vi "Test Server API.vi"() -> ()   [LabVIEW 2019]
doc: "Server API Tester."
uses:
  TypeDef/ISO.ctl
  TypeDef/Noise.ctl
  TypeDef/Link.ctl
  TypeDef/Sett data.ctl
  Server.lvlib
  Setting Panel/Setting Panel.lvlib
panel:
  out "Distance 2":dbl
  out "Signal gain 2":dbl
  out "Noise attenuator 2":dbl
  out "Link 2":T1
  out "Type noise 2":T2
  out "M 2":cluster{"Метка":i64, "Считыветель":i64}
  out "BM 3":cluster{"R":dbl, "C":dbl, "L":dbl}
  out "BI 3":cluster{"R":dbl, "C":dbl, "L":dbl}
  out "ISO/IEC w 2":T3
  out "Bit rate 3":dbl
  out "Gain 2":dbl
  out "Filter 3":i32
  out "Distance":dbl
  out "Signal gain":dbl
  out "Noise attenuator":dbl
  out "Link":T1
  out "Type noise":T2
  out "M":cluster{"Метка":i64, "Считыветель":i64}
  out "BM 2":cluster{"R":dbl, "C":dbl, "L":dbl}
  out "BI 2":cluster{"R":dbl, "C":dbl, "L":dbl}
  out "ISO/IEC w":T3
  out "Bit rate 2":dbl
  out "Gain":dbl
  out "Filter 2":i32
  in  "Bit rate":dbl=32.0 min=4.0 max=128.0 step=4.0
  in  "Filter":i32=3 min=1 max=15 step=1
  in  "Type noise w":T2
  in  "M w":cluster{"Метка":i64, "Считыветель":i64}={"Метка"=10, "Считыветель"=100} {"Считыветель" min=10 max=10 step=100; "Метка" min=10 max=10 step=100}
  in  "BM":cluster{"R":dbl, "C":dbl, "L":dbl}={"R"=1.0, "C"=0.01, "L"=1e-05} {"L" min=1e-05 max=1.5e-05 step=1e-06 format="%#_6p"; "C" min=0.01 max=0.15 step=0.001 format="%#_6p"; "R" min=1.0 max=150.0 step=1.0 format="%#_6p"}
  in  "BI":cluster{"R":dbl, "C":dbl, "L":dbl}={"R"=1.0, "C"=0.01, "L"=1e-05} {"L" min=1e-05 max=1.5e-05 step=1e-06 format="%#_6p"; "C" min=0.01 max=0.15 step=0.001 format="%#_6p"; "R" min=1.0 max=150.0 step=1.0 format="%#_6p"}
  in  "Иммитатор расстояния":dbl(slide)=3.0 min=3.0 max=1500.0 step=1.0 scale=3.0..1500.0
  in  "Усилитель сигнала":dbl(knob)=1.0 min=1.0 max=100.0 step=1.0 scale=1.0..30.0
  in  "Выбор стандарта":T3
  in  "Аттенюатор шума":dbl(knob)=1.0 min=1.0 max=10.0 step=0.1 scale=1.0..30.0
  in  "Apply Settings":bool
  in  "wait for reply":bool=TRUE
  in  "Show Block Diagram":bool
  in  "X":dbl=1.0
  out "Reply Payload":dbl
  in  "Stop Module":bool
  in  "Start Module":bool
  out "Do Something Count":i32
  in  "Test Do Something Else and Wait for Reply":bool
  in  "Hide Module Panel":bool
  in  "Show Module Panel":bool
  in  "Test Do Something Else":bool
  in  "Start":bool
  out "Status":string
  out "Module Running?":bool
  # "Данные отправляемые в модуль"
  # "Данные из модуля\n Settings"
  # "При нажатии кнопки Apply на лицевой\nпанели модуля Server"
  # "This VI tests the API for the Module."
  # "БУПУЭМСС"
  # "БУПУЭМСМ"
  # "Коэффициент модуляции, %"
  # "Скорость"
  # "Порядок фильтра"
  # "Для отправления данных в модули\nработчих каналов"
  # "мм"
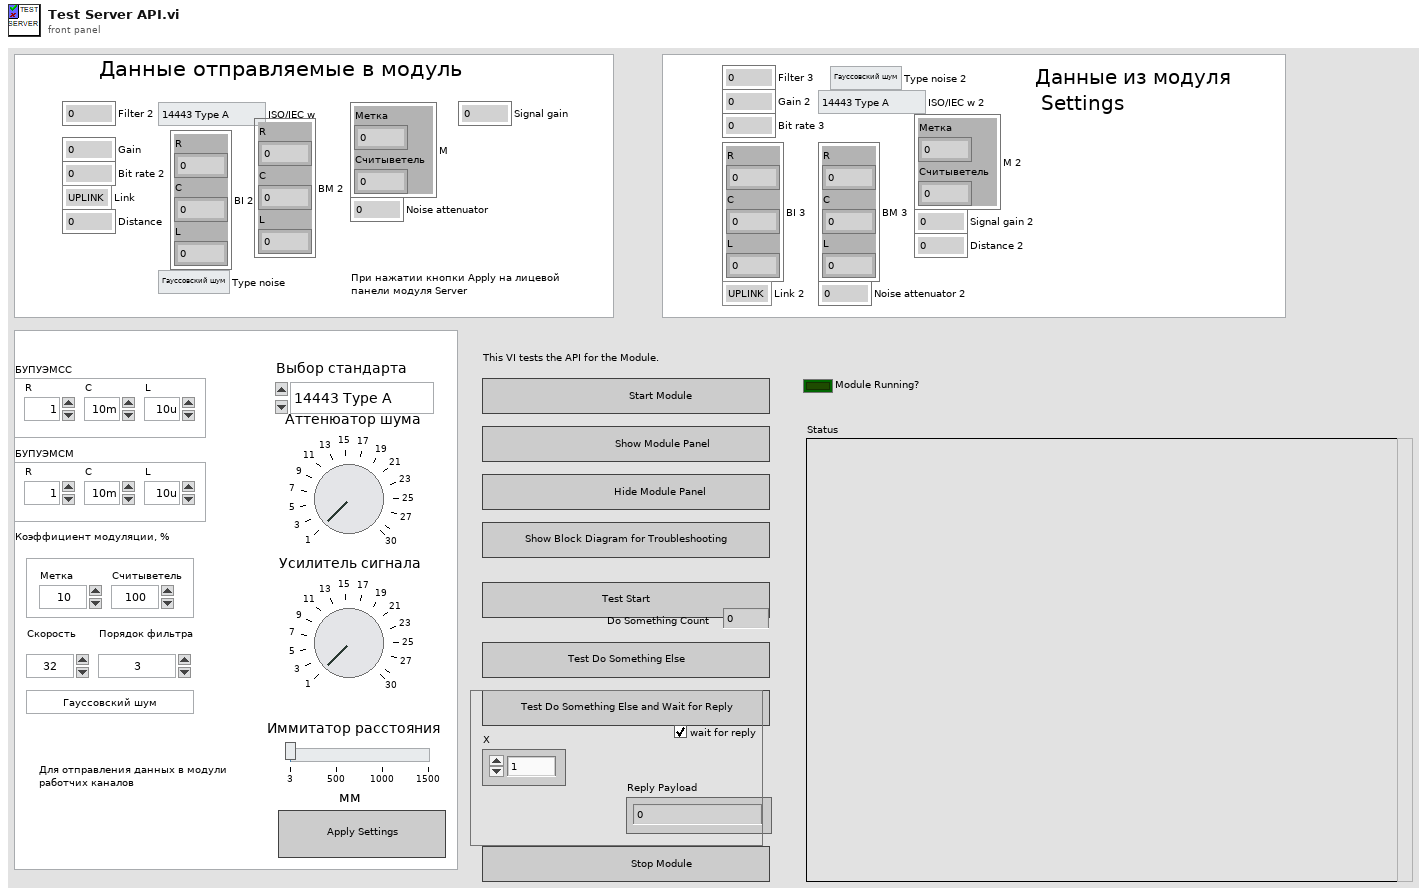
[diagram p1: front panel]
types:
  T1 = typedef "Link.ctl" = enum16{"UPLINK", "DOWNLINK"}
  T2 = typedef "Noise.ctl" = enum16{"Гауссовский шум", "Белый шум"}
  T3 = typedef "ISO.ctl" = enum16{"14443 Type A", "14443 Type B", "Felica", "15693"}
  T4 = typedef "Server.lvlib/Broadcast Events--cluster.ctl" = cluster{"Module Did Init":refnum<user-event>, "Status Updated":refnum<user-event>, "Error Reported":refnum<user-event>, "Did Something":refnum<user-event>, "Module Did Stop":refnum<user-event>, "Update Module Execution Status":refnum<user-event>, "Apply settings":refnum<user-event>}
  T5 = typedef "Setting Panel.lvlib/Broadcast Events--cluster.ctl" = cluster{"Module Did Init":refnum<user-event>, "Status Updated":refnum<user-event>, "Error Reported":refnum<user-event>, "Did Something":refnum<user-event>, "Module Did Stop":refnum<user-event>, "Update Module Execution Status":refnum<user-event>, "Get data":refnum<user-event>}
  T6 = typedef "Sett data.ctl" = cluster{"Filter":i32, "Gain":dbl, "Bit rate":dbl, "ISO/IEC w ":T3, "BI":cluster{"R":dbl, "C":dbl, "L":dbl}, "BM":cluster{"R":dbl, "C":dbl, "L":dbl}, "M":cluster{"Метка":i64, "Считыветель":i64}, "Type noise":T2, "Link":T1, "Noise attenuator":dbl, "Signal gain":dbl, "Distance":dbl}
  T7 = typedef "Server.lvlib/Do Something Else and Wait (Reply Payload)--cluster.ctl" = cluster{"Value":dbl, "error":errorcluster}
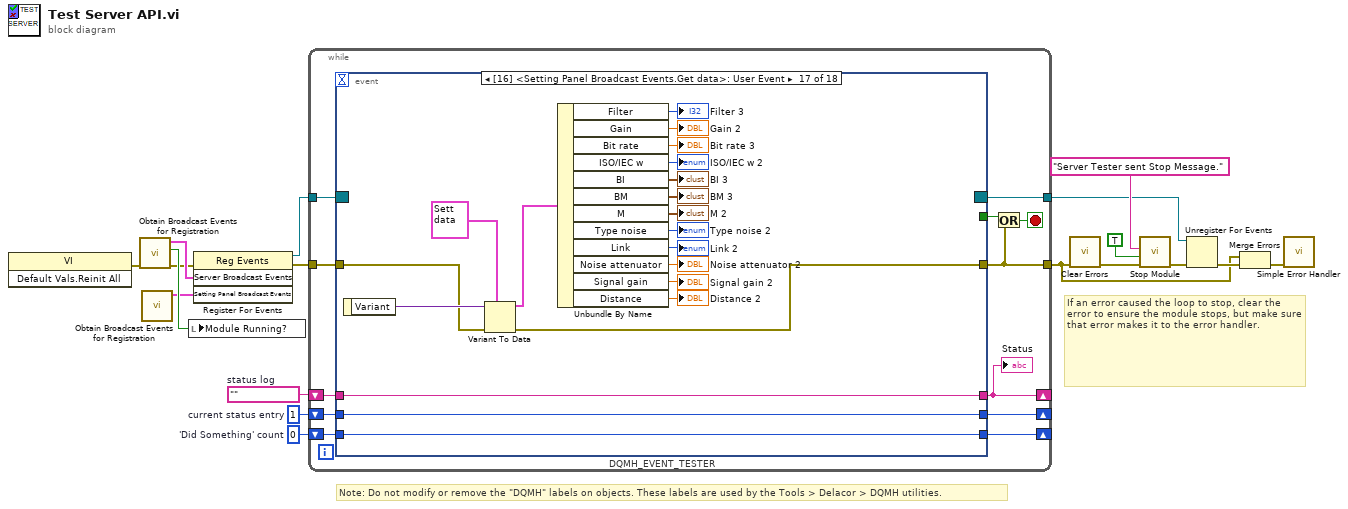
[diagram p0: block diagram]
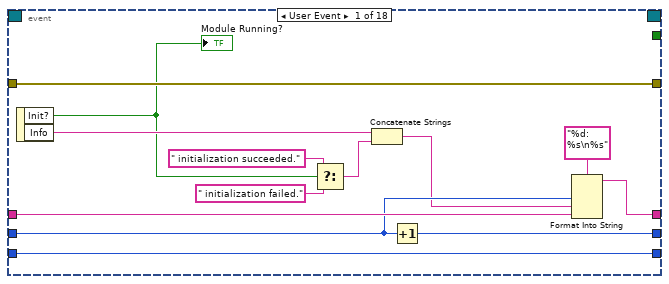
[diagram p2: hidden frame]
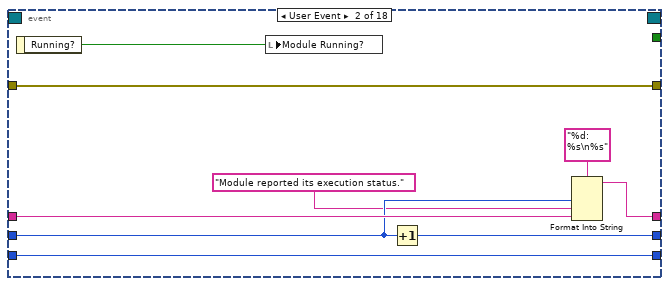
[diagram p3: hidden frame]
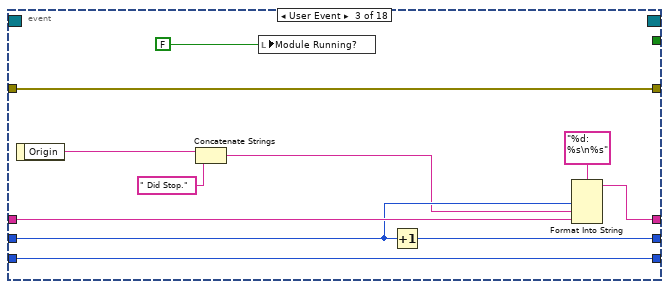
[diagram p4: hidden frame]
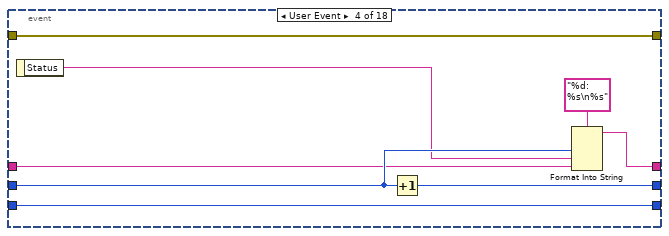
[diagram p5: hidden frame]
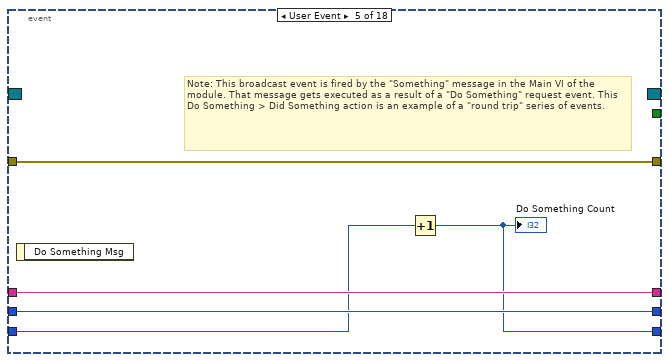
[diagram p6: hidden frame]
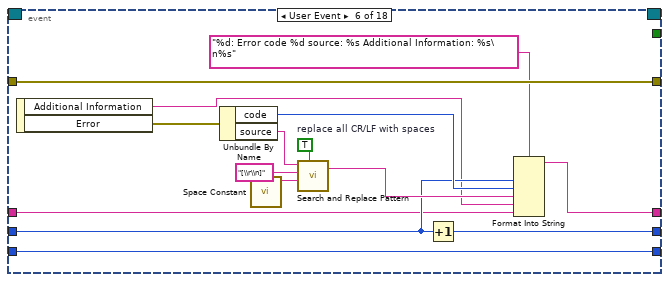
[diagram p7: hidden frame]
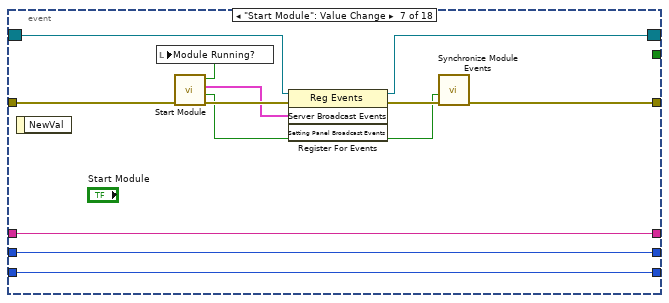
[diagram p8: hidden frame]
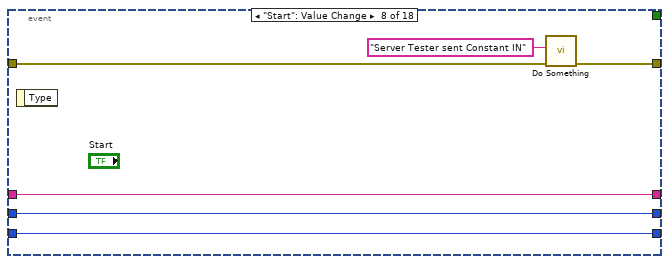
[diagram p9: hidden frame]
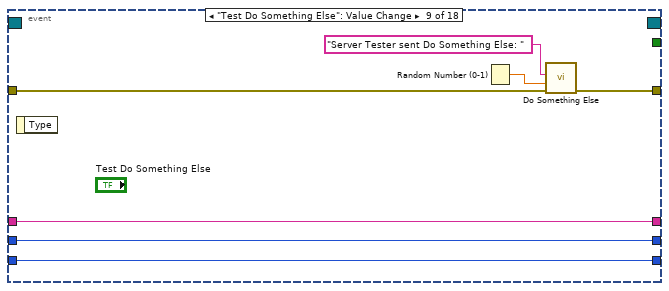
[diagram p10: hidden frame]
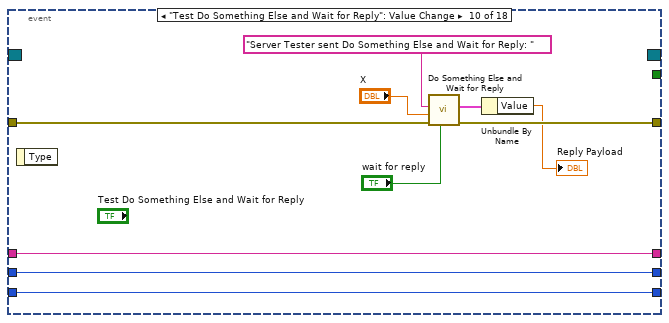
[diagram p11: hidden frame]
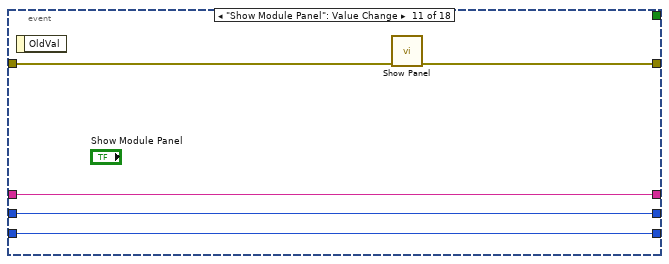
[diagram p12: hidden frame]
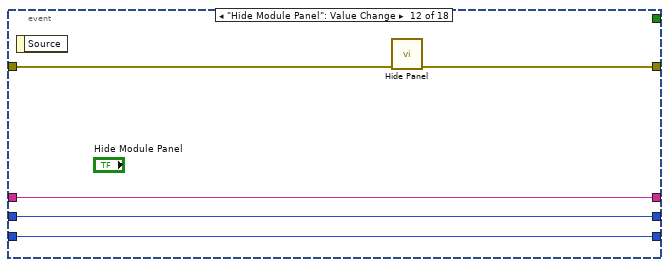
[diagram p13: hidden frame]
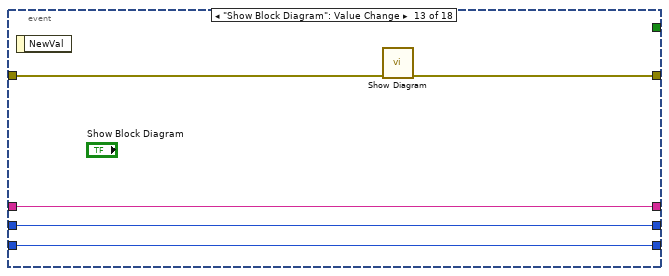
[diagram p14: hidden frame]
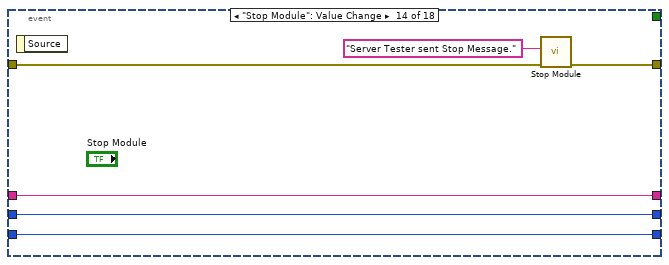
[diagram p15: hidden frame]
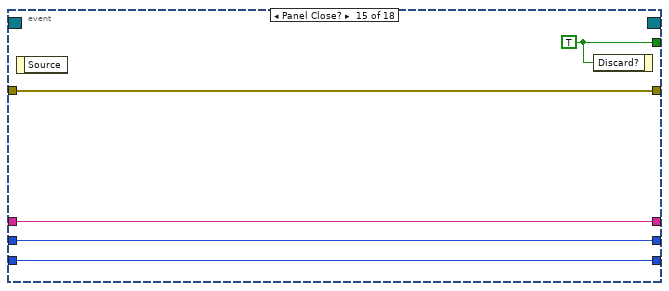
[diagram p16: hidden frame]
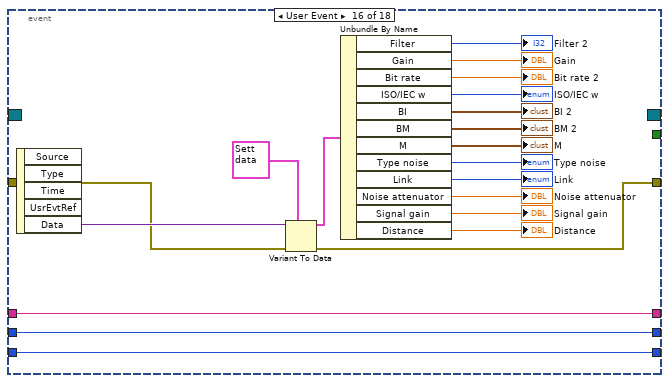
[diagram p17: hidden frame]
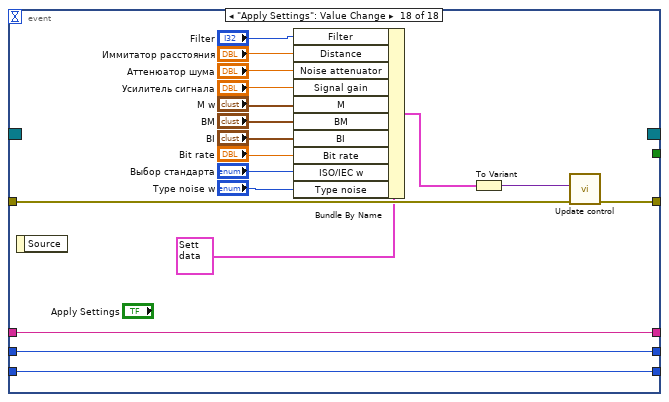
[diagram p18: hidden frame]
diagram:
  w13 = 0  # 'Did Something' count
  w14 = 1  # current status entry
  w15 = ""  # status log
  # "If an error caused the loop to stop, clear the error to ensure the module stops, but make sure that error makes it to the error handler."
  # "Note: Do not modify or remove the \"DQMH\" labels on objects. These labels are used by the Tools > Delacor > DQMH utilities."
  n1 = invoke class="VI" method="Default Vals.Reinit All"() -> (error out=w3:errorcluster)  [unwired: 3 in, 2 out]
  n2 = call "Obtain Broadcast Events for Registration.vi"("error in (no error)"=w3) -> ("error out"=w2:errorcluster, "Already running?"=w4:bool, "Server Broadcast Events"=w11:T4)  [unwired: 8 in]
  n3 = call "Obtain Broadcast Events for Registration.vi"() -> ("Setting Panel Broadcast Events"=w1:T5)  [unwired: 9 in, 2 out]
  n4 = local write "Module Running?"(w4) -> ()
  n5 = register-events(error in=w2, w11, w1) -> (reference out=w10:refnum<event-registration>, error out=w12:errorcluster)  [unwired: 1 in]
  n6 = while {
    tunnel: w10 -> [w30]
    tunnel: [w19] -> w5
    shift-right: [w25] -> _
    shift-left: w15 -> [w27]
    shift-right: [w26] -> _
    shift-left: w14 -> [w28]
    shift-right: [w23] -> _
    shift-left: w13 -> [w24]
    tunnel: w12 -> [w21]
    tunnel: [w20] -> w9
    stop <- w22 stop-if-true
    n7 = event "DQMH_EVENT_TESTER" shown="[16] <Setting Panel Broadcast Events.Get data>: User Event" {
      selector: w30 -> [_ _ _ _ _ _ w96 _ _ _ _ _ _ _ _ _ _ _]
      dyn-events: [_ _ _ _ _ _ w95 _ _ _ _ _ _ _ _ _ _ _] -> w20
      timeout: _ -> [_ _ _ _ _ _ _ _ _ _ _ _ _ _ _ _ _ _]
      tunnel: [_ _ _ _ _ _ _ _ _ _ _ _ _ _ w152 _ _ _] -> w29
      tunnel: [w43 w45 w53 w64 w72 w90 w94 w109 w116 w126 w131 w136 w137 w144 w148 w167 w187 w206] -> w19
      tunnel: w28 -> [w40 w50 w61 w68 w75 w80 w100 w106 w112 w123 w129 w134 w139 w146 w150 w171 w191 w208]
      tunnel: w27 -> [w41 w51 w62 w67 w76 w78 w101 w107 w113 w124 w130 w135 w140 w147 w151 w172 w192 w209]
      tunnel: [w38 w48 w59 w69 w76 w81 w101 w107 w113 w124 w130 w135 w140 w147 w151 w172 w192 w209] -> w25
      tunnel: [w39 w49 w60 w71 w75 w79 w100 w106 w112 w123 w129 w134 w139 w146 w150 w171 w191 w208] -> w26
      tunnel: w24 -> [w35 w46 w55 w65 w74 w91 w99 w105 w111 w122 w128 w133 w138 w145 w149 w170 w190 w207]
      tunnel: [w35 w46 w55 w65 w73 w91 w99 w105 w111 w122 w128 w133 w138 w145 w149 w170 w190 w207] -> w23
      tunnel: w21 -> [w43 w45 w53 w64 w72 w90 w93 w104 w110 w119 w127 w132 w141 w142 w148 w168 w188 w210]
      event User Event {
        n8 = event-data() -> ("Init?"=w34:bool, "Info"=w37:string)  [unwired: 1 in]
        "Module Running?" <- w34
        n9 = Select(t=" initialization succeeded.", s=w34, f=" initialization failed.") -> (s? t:f=w31:string)
        n10 = Concatenate Strings(w37, w31) -> (w36:string)
        n11 = Increment(x=w40) -> (x+1=w39:i32)
        n12 = Format Into String(format string="%d: %s\n%s", w40, w36, w41) -> (resulting string=w38:string)  [unwired: 2 in, 1 out]
      }
      event User Event {
        n13 = event-data() -> ("Running?"=w44:bool)  [unwired: 1 in]
        n14 = local write "Module Running?"(w44) -> ()
        n15 = Increment(x=w50) -> (x+1=w49:i32)
        n16 = Format Into String(format string="%d: %s\n%s", w50, "Module reported its execution status.", w51) -> (resulting string=w48:string)  [unwired: 2 in, 1 out]
      }
      event User Event {
        n17 = event-data() -> ("Origin"=w58:string)  [unwired: 1 in]
        n18 = Concatenate Strings(w58, " Did Stop.") -> (w57:string)
        n19 = local write "Module Running?"(FALSE ("Module Did Init?")) -> ()
        n20 = Increment(x=w61) -> (x+1=w60:i32)
        n21 = Format Into String(format string="%d: %s\n%s", w61, w57, w62) -> (resulting string=w59:string)  [unwired: 2 in, 1 out]
      }
      event User Event {
        n22 = event-data() -> ("Status"=w66:string)  [unwired: 1 in]
        n23 = Increment(x=w68) -> (x+1=w71:i32)
        n24 = Format Into String(format string="%d: %s\n%s", w68, w66, w67) -> (resulting string=w69:string)  [unwired: 2 in, 1 out]
      }
      event User Event {
        # "Note: This broadcast event is fired by the \"Something\" message in the Main VI of the module. That message gets executed as a result of a \"Do Something\" request event. This Do Something > Did Something action is an example of a \"round trip\" series of events."
        n25 = event-data() -> ()  [unwired: 1 in, 1 out]
        n26 = Increment(x=w74) -> (x+1=w73:i32)
        "Do Something Count" <- w73
      }
      event User Event {
        w86 = TRUE  # replace all CR/LF with spaces
        n27 = event-data() -> ("Additional Information"=w77:string, "Error"=w82:errorcluster)  [unwired: 1 in]
        n28 = Unbundle By Name(w82) -> ("code"=w83:i32, "source"=w84:string)
        n29 = call <vilib>:"Space Constant.vi"() -> ("String"=w87:string)
        n30 = call <vilib>:"Search and Replace Pattern.vi"("string"=w84, "regular expression (\"\")"="[\\r\\n]" ("regular expression (\"\")"), "replace string (\"\")"=w87, "replace all? (F)"=w86) -> ("result string"=w85:string)  [unwired: 1 in, 1 out]
        n31 = Increment(x=w80) -> (x+1=w79:i32)
        n32 = Format Into String(format string="%d: Error code %d source: %s Additional Information: %s\n%s", w80, w83, w85, w77, w78) -> (resulting string=w81:string)  [unwired: 2 in, 1 out]
      }
      event "Start Module": Value Change {
        n33 = event-data() -> ()  [unwired: 1 in, 1 out]
        n34 = call "Start Module.vi"("error in (no error)"=w93) -> ("error out"=w102:errorcluster, "Wait for Event Sync?"=w98:bool, "Server Broadcast Events"=w97:T4, "Module Was Already Running?"=w92:bool)  [unwired: 7 in]
        n35 = local write "Module Running?"(w92) -> ()
        n36 = register-events(reference=w96, error in=w102, w97) -> (reference out=w95:refnum<event-registration>, error out=w103:errorcluster)  [unwired: 1 in]
        n37 = call "Synchronize Module Events.vi"("error in (no error)"=w103, "Wait for Event Sync?"=w98) -> ("error out"=w94:errorcluster)  [unwired: 9 in]
      }
      event "Start": Value Change {
        n38 = event-data() -> ()  [unwired: 1 in, 1 out]
        n39 = call "Do Something.vi"("error in (no error)"=w104, "Do Something Message"="Server Tester sent Constant IN") -> ("error out"=w109:errorcluster)  [unwired: 9 in]
      }
      event "Test Do Something Else": Value Change {
        n40 = event-data() -> ()  [unwired: 1 in, 1 out]
        n41 = Random Number (0-1)() -> (number: 0 to 1=w114:dbl)
        n42 = call "Do Something Else.vi"("error in (no error)"=w110, "X"=w114, "Do Something Else Message"="Server Tester sent Do Something Else: " ("Do Something Message")) -> ("error out"=w116:errorcluster)  [unwired: 8 in]
      }
      event "Test Do Something Else and Wait for Reply": Value Change {
        n43 = event-data() -> ()  [unwired: 1 in, 1 out]
        n44 = call "Do Something Else and Wait for Reply.vi"("wait for reply (T)"="wait for reply", "error in (no error)"=w119, "X"="X", "Do Something Else Message"="Server Tester sent Do Something Else and Wait for Reply: " ("Do Something Message")) -> ("error out"=w126:errorcluster, "Reply Payload"=w121:T7)  [unwired: 5 in, 1 out]
        n45 = Unbundle By Name(w121) -> ("Value"=→"Reply Payload":dbl)
      }
      event "Show Module Panel": Value Change {
        n46 = event-data() -> ()  [unwired: 1 in, 1 out]
        n47 = call "Show Panel.vi"("error in (no error)"=w127) -> ("error out"=w131:errorcluster)  [unwired: 10 in]
      }
      event "Hide Module Panel": Value Change {
        n48 = event-data() -> ()  [unwired: 1 in, 1 out]
        n49 = call "Hide Panel.vi"("error in (no error)"=w132) -> ("error out"=w136:errorcluster)  [unwired: 10 in]
      }
      event "Show Block Diagram": Value Change {
        n50 = event-data() -> ()  [unwired: 1 in, 1 out]
        n51 = call "Show Diagram.vi"("error in (no error)"=w141) -> ("error out"=w137:errorcluster)  [unwired: 10 in]
      }
      event "Stop Module": Value Change {
        n52 = event-data() -> ()  [unwired: 1 in, 1 out]
        n53 = call "Stop Module.vi"("error in (no error)"=w142, "Origin"="Server Tester sent Stop Message.") -> ("error out"=w144:errorcluster)  [unwired: 9 in]
      }
      event Panel Close? {
        w152 = TRUE ("Discard?")
        n54 = event-data() -> ()  [unwired: 1 in, 1 out]
        n55 = event-data("Discard?"=w152) -> ()  [unwired: 1 in, 1 out]
      }
      event User Event {
        n56 = event-data() -> ("Data"=w169:variant)  [unwired: 1 in, 4 out]
        n57 = Variant To Data(error in=w168, type=T6 {"Filter"=0, "Gain"=0.0, "Bit rate"=0.0, "ISO/IEC w "=enum."14443 Type A", "BI"={"R"=0.0, "C"=0.0, "L"=0.0}, "BM"={"R"=0.0, "C"=0.0, "L"=0.0}, "M"={"Метка"=10, "Считыветель"=10}, "Type noise"=enum."Гауссовский шум", "Link"=enum."UPLINK", "Noise attenuator"=0.0, "Signal gain"=1.0, "Distance"=0.0} ("Sett data"), Variant=w169) -> (data=w165:T6, error out=w167:errorcluster)
        n58 = Unbundle By Name(w165) -> ("Filter"=→"Filter 2":i32, "Gain"=→"Gain":dbl, "Bit rate"=→"Bit rate 2":dbl, "ISO/IEC w"=→"ISO/IEC w":T3, "BI"=→"BI 2":cluster{"R":dbl, "C":dbl, "L":dbl}, "BM"=→"BM 2":cluster{"R":dbl, "C":dbl, "L":dbl}, "M"=→"M":cluster{"Метка":i64, "Считыветель":i64}, "Type noise"=→"Type noise":T2, "Link"=→"Link":T1, "Noise attenuator"=→"Noise attenuator":dbl, "Signal gain"=→"Signal gain":dbl, "Distance"=→"Distance":dbl)
      }
      event User Event {
        n59 = event-data() -> ("Variant"=w189:variant)  [unwired: 1 in]
        n60 = Variant To Data(error in=w188, type=T6 {"Filter"=0, "Gain"=0.0, "Bit rate"=0.0, "ISO/IEC w "=enum."14443 Type A", "BI"={"R"=0.0, "C"=0.0, "L"=0.0}, "BM"={"R"=0.0, "C"=0.0, "L"=0.0}, "M"={"Метка"=10, "Считыветель"=10}, "Type noise"=enum."Гауссовский шум", "Link"=enum."UPLINK", "Noise attenuator"=0.0, "Signal gain"=1.0, "Distance"=0.0} ("Sett data"), Variant=w189) -> (data=w185:T6, error out=w187:errorcluster)
        n61 = Unbundle By Name(w185) -> ("Filter"=→"Filter 3":i32, "Gain"=→"Gain 2":dbl, "Bit rate"=→"Bit rate 3":dbl, "ISO/IEC w"=→"ISO/IEC w 2":T3, "BI"=→"BI 3":cluster{"R":dbl, "C":dbl, "L":dbl}, "BM"=→"BM 3":cluster{"R":dbl, "C":dbl, "L":dbl}, "M"=→"M 2":cluster{"Метка":i64, "Считыветель":i64}, "Type noise"=→"Type noise 2":T2, "Link"=→"Link 2":T1, "Noise attenuator"=→"Noise attenuator 2":dbl, "Signal gain"=→"Signal gain 2":dbl, "Distance"=→"Distance 2":dbl)
      }
      event "Apply Settings": Value Change {
        n62 = event-data() -> ()  [unwired: 1 in, 1 out]
        n63 = Bundle By Name(cluster=T6 {"Filter"=0, "Gain"=0.0, "Bit rate"=0.0, "ISO/IEC w "=enum."14443 Type A", "BI"={"R"=0.0, "C"=0.0, "L"=0.0}, "BM"={"R"=0.0, "C"=0.0, "L"=0.0}, "M"={"Метка"=10, "Считыветель"=10}, "Type noise"=enum."Гауссовский шум", "Link"=enum."UPLINK", "Noise attenuator"=0.0, "Signal gain"=1.0, "Distance"=0.0} ("Sett data"), "Filter"="Filter", "Distance"="Иммитатор расстояния", "Noise attenuator"="Аттенюатор шума", "Signal gain"="Усилитель сигнала", "M"="M w", "BM"="BM", "BI"="BI", "Bit rate"="Bit rate", "ISO/IEC w"="Выбор стандарта", "Type noise"="Type noise w") -> (w204:T6)
        n64 = To Variant(anything=w204) -> (Variant=w203:variant)
        n65 = call "Update control.vi"("error in (no error)"=w210, "Variant"=w203) -> ("error out"=w206:errorcluster)  [unwired: 9 in]
      }
    }
    "Status" <- w25
    n66 = Or(x=w29, y=w19) -> (x .or. y?=w22:bool)
  }
  n67 = call <vilib>:"Clear Errors.vi"("error in (no error)"=w5) -> ("error out"=w7:errorcluster)  [unwired: 5 in, 1 out]
  n68 = call "Stop Module.vi"("error in (no error)"=w7, "Wait for Module to Stop? (F)"=TRUE ("Wait for Module to stop?"), "Origin"="Server Tester sent Stop Message.") -> ("error out"=w17:errorcluster)  [unwired: 8 in]
  n69 = Unregister For Events(event registration refnum=w9, error in=w17) -> (error out=w18:errorcluster)
  n70 = Merge Errors(w5, w18) -> (w6:errorcluster)
  n71 = call <vilib>:"Simple Error Handler.vi"("error in (no error)"=w6) -> ()  [unwired: 4 in, 5 out]
